vi "Teleop.vi"(10 "Match Info":T2={"Autonomous Elapsed Seconds"=0.0, "TeleOp Elapsed Seconds"=33.944, "Disabled Elapsed Seconds"=47.199, "Visited Autonomous"=FALSE, "Visited TeleOp"=TRUE, "Visited Disabled"=TRUE, "Autonomous Settings"={"Autonomous Style"=enum."Independent", "VI Refnum"=refnum}}, 11 "Call Context":T3=enum."Stop") -> ()   [LabVIEW 2017]
doc: "This VI is called for each enabled TeleOp packet received from the DS. It is typically used to read from joysticks and other inputs and update I/O or setpoints for timed control loops. It should complete and return within 20 milliseconds or risk missing DS packets."
uses:
  <vilib>/Rock Robotics/WPI/DriverStation/WPI_DriverStationDerivedRobotMode.ctl
  <vilib>/Rock Robotics/WPI/DriverStation/WPI_DriverStationMatch Info.ctl
  <vilib>/Rock Robotics/WPI/Utilities/WPI_GetSetVariantRefNum.vi
  <vilib>/Rock Robotics/Network Tables/NT Write Boolean Array.vi
  <vilib>/Rock Robotics/Network Tables/NT Write Numeric Array.vi
  Framework/Robot Global Data.vi
panel:
  out "Gyro Angle":dbl=359.5340095519775
  out "Angle":dbl(knob)=359.5340095519775 scale=0.0..360.0
  in  "Dead Zone(0 to 1)":dbl=0.01
  in  "Enum":T1(ring)=enum."Square"
  in  "n^x(Unbounded)":dbl=2.5 format="%#_13g"
  in  "Min Output(0 to 1)":dbl=0.01
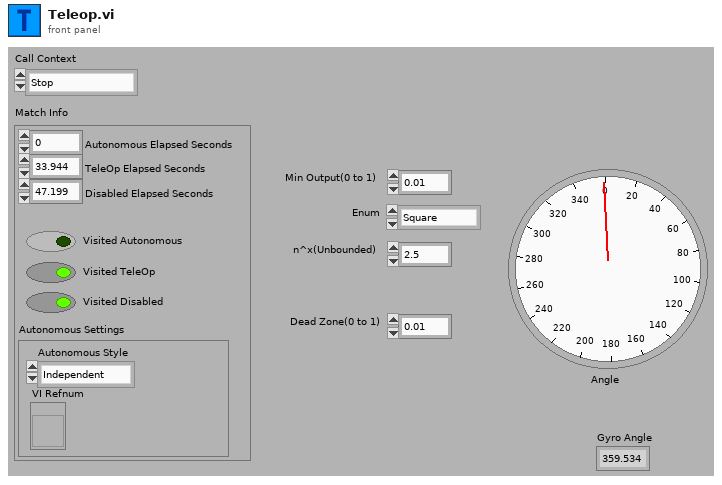
[diagram p1: front panel]
types:
  T1 = enum16{"Linear", "Square  Root", "Square", "n^x"}
  T2 = typedef "WPI_DriverStationMatch Info.ctl" = cluster{"Autonomous Elapsed Seconds":dbl, "TeleOp Elapsed Seconds":dbl, "Disabled Elapsed Seconds":dbl, "Visited Autonomous":bool, "Visited TeleOp":bool, "Visited Disabled":bool, "Autonomous Settings":cluster{"Autonomous Style":enum16{"Iterative", "Independent"}, "VI Refnum":refnum<vi>}}
  T3 = typedef "WPI_DriverStationDerivedRobotMode.ctl" = enum16{"Init", "Execute", "Stop"}
  T4 = typedef "WPI_JoystickDevRef.ctl" = cluster{"Device":T5}
  T5 = typedef "WPI_JoystickDeviceEnum.ctl" = enum16{"USB 0", "USB 1", "USB 2", "USB 3", "USB 4", "USB 5"}
  T6 = cluster{"X":dbl, "Y":dbl, "Angle":dbl, "Magnitude":dbl}
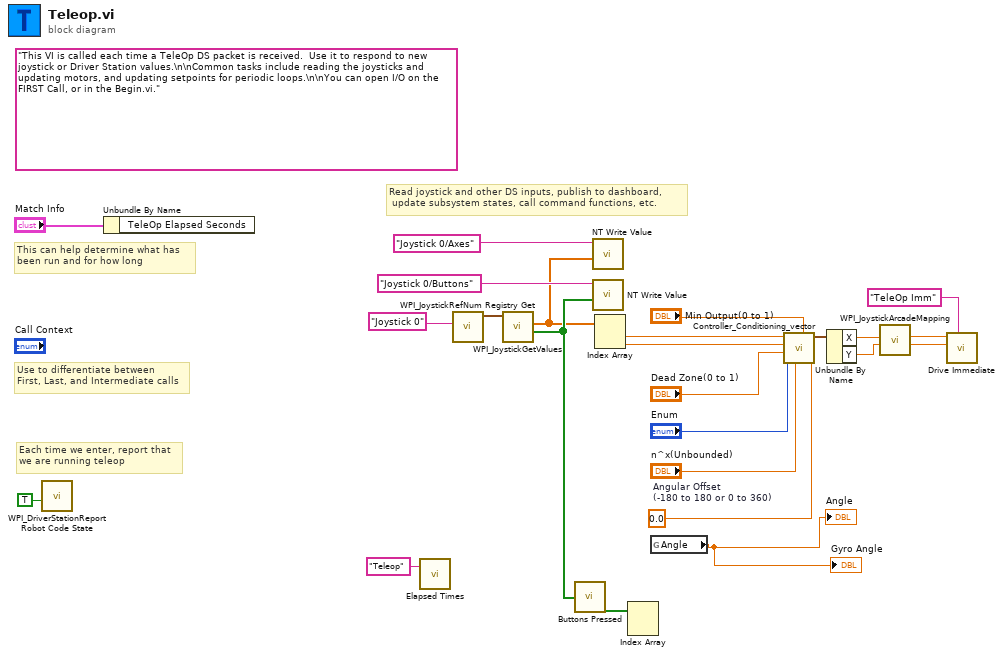
[diagram p0: block diagram]
diagram:
  w3 = 0.0  # Angular Offset (-180 to 180 or 0 to 360)
  (unwired) "This VI is called each time a TeleOp DS packet is received.  Use it to respond to new joystick or Driver Station values.\n\nCommon tasks include reading the joysticks and updating motors, and updating setpoints for periodic loops.\n\nYou can open I/O on the FIRST Call, or in the Begin.vi."
  # "Read joystick and other DS inputs, publish to dashboard,\n update subsystem states, call command functions, etc."
  # "Each time we enter, report that\nwe are running teleop"
  # "Use to differentiate between\nFirst, Last, and Intermediate calls"
  # "This can help determine what has\nbeen run and for how long"
  n1 = call <vilib>:"WPI_DriverStationReport Robot Code State.vi"("TeleOp"=TRUE ("Autonomous")) -> ()  [unwired: 10 in, 1 out]
  n2 = Unbundle By Name("Match Info") -> ()  [unwired: 1 out]
  n3 = call "Elapsed Times.vi"("Call Name"="Teleop") -> ()  [unwired: 2 in, 1 out]
  n4 = call <vilib>:"WPI_JoystickRefNum Registry Get.vi"("refnum name"="Joystick 0") -> ("JoystickDevRef"=w21:T4)  [unwired: 1 in, 9 out]
  n5 = call <vilib>:"WPI_JoystickGetValues.vi"("JoystickDevRef"=w21) -> ("Buttons"=w15:bool[], "Axes"=w14:dbl[])  [unwired: 6 in, 3 out]
  n6 = call "Buttons Pressed.vi"("Button Values"=w15) -> ("Button Presses"=w19:bool[])
  n7 = call-poly <vilib>:"NT Write Value.vi"("Numeric Array"=w14, "Name"="Joystick 0/Axes") -> ()  [unwired: 9 in, 1 out]
  n8 = call-poly <vilib>:"NT Write Value.vi"("Boolean Array"=w15, "Name"="Joystick 0/Buttons") -> ()  [unwired: 9 in, 1 out]
  n9 = Index Array(array=w14) -> (element #1=w8:dbl, element #2=w7:dbl)  [unwired: 2 in]
  n10 = Index Array(array=w19) -> ()  [unwired: 2 in, 2 out]
  n11 = global read "Robot Global Data.vi" "Angle"() -> (→"Angle" →"Gyro Angle":dbl)
  n12 = call "Controller_Conditioning_vector.vi"("Angular Offset\n(-180 to 180 or 0 to 360)"=w3, "Min Output(0 to 1)"="Min Output(0 to 1)", "n^x(Unbounded)"="n^x(Unbounded)", "Enum"="Enum", "Dead Zone(0 to 1)"="Dead Zone(0 to 1)", "Y(-1 to 1)"=w7, "X(-1 to 1)"=w8) -> ("output cluster"=w6:T6)  [unwired: 4 in]
  n13 = Unbundle By Name(w6) -> ("X"=w5:dbl, "Y"=w4:dbl)
  n14 = call <vilib>:"WPI_JoystickArcadeMapping.vi"("Y axis value"=w4, "X axis value"=w5) -> ("Right Motor Value"=w17:dbl, "Left Motor Value"=w18:dbl)  [unwired: 8 in]
  n15 = call "Drive Immediate.vi"("Description"="TeleOp Imm", "Right Setpoint"=w17, "Left Setpoint"=w18) -> ()  [unwired: 8 in, 1 out]
